vi "getArrowHead.vi"(0 "reference":refnum<class "ArrowHead.lvclass">, 5 "error in (no error)":errorcluster) -> (14 "reference out":refnum<class "ArrowHead.lvclass">, 15 "arrowHead":T1, 19 "error out":errorcluster)   [LabVIEW 2020, in "ArrowHead.lvclass"]
doc: "Gets the arrow head type"
uses:
  <resource>/Framework/Providers/Open_GDS/UML/ArrowHead_class/ArrowHead.lvclass
  <resource>/Framework/Providers/Open_GDS/UML/ArrowHead_class/ArrowHeadType.ctl
  <resource>/Framework/Providers/Open_GDS/UML/ArrowHead_class/ArrowHead.lvclass/ArrowHead.ctl
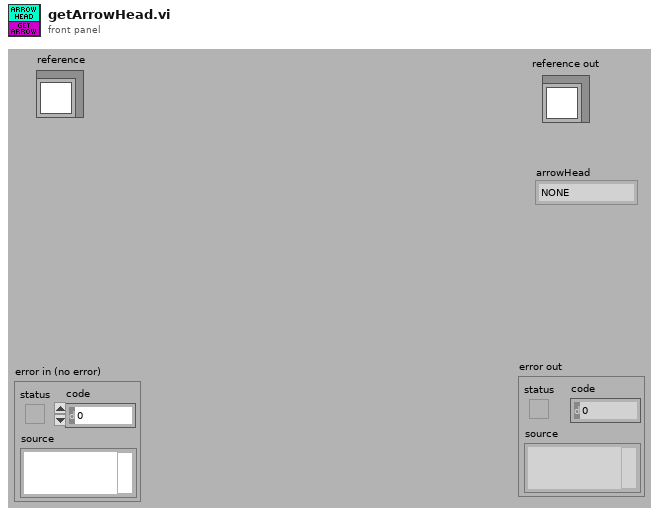
[diagram p1: front panel]
types:
  T1 = typedef "ArrowHead.lvclass/ArrowHeadType.ctl" = enum16{"NONE", "TRIANGLE", "BLACK_TRIANGLE", "V", "HALF_V", "DIAMOND", "BLACK_DIAMOND"}
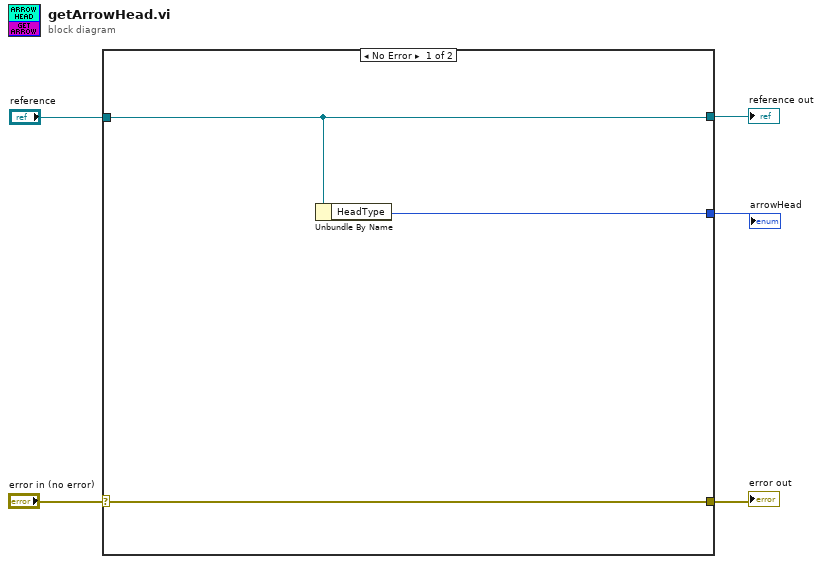
[diagram p0: block diagram]
diagram:
  n1 = case shown="No Error" "error in (no error)" {
    selector: "error in (no error)" -> [w7 w9]
    tunnel: "reference" -> [w8 w10]
    tunnel: [w7 w9] -> w3
    tunnel: [w8 w10] -> w2
    tunnel: [w6 _] -> w1
    frame No Error {
      n2 = Unbundle By Name(w8) -> ("HeadType"=w6:T1)
    }
    frame Error {
    }
  }
  "reference out" <- w2
  "error out" <- w3
  "arrowHead" <- w1
